vi "ShowZLUTBias.vi"(11 "Bias planes":i32) -> ()   [LabVIEW 2011]
uses:
  Main/GlobalVariables.vi
panel:
  in  "Bead index":i32
  out "Bias":sgl[](graph)
  out "All beads bias":sgl[][](graph)
  in  "Close dialog":bool
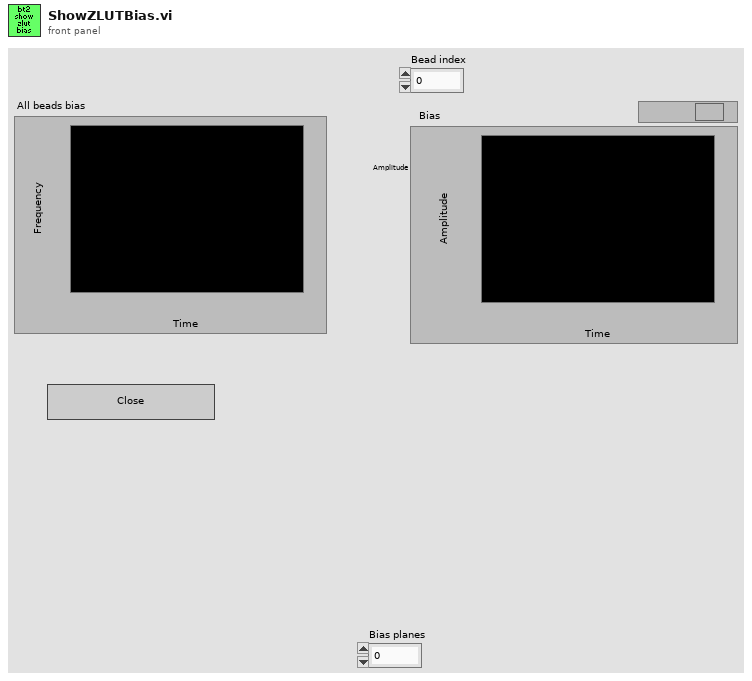
[diagram p1: front panel]
types:
  T1 = typedef "MeasureConfigType.ctl" = cluster{"Bead locations":cluster{"X":i32, "Y":i32}[], "ROI":i32, "Experiment base path":path, "Image output subdir":string, "Output mode":T2, "Traces output subdir":string, "QTrk Settings":T3, "Tracking Config":T4, "Experiment Name":string, "Program":T7, "ZLUT":sgl[][][], "Camera settings":T14, "Experiment Script":string, "Max frames in memory":i32, "Save traces as binary":bool, "Pixel Calibration Gain Image":string, "Pixel Calibration Offset Image":string, "Use pixel calibration images":bool, "Internal camera settings":string, "Trace write interval":i32}
  T2 = typedef "MeasureConfigOutputMode.ctl" = enum16{"None", "Track", "SaveImages"}
  T3 = typedef "QTrkSettings.ctl" = cluster{"Image width":i32, "Image height":i32, "Number of threads (CPU based)":i32, "CUDA Device":i32, "COM Background correction factor":sgl, "ZLUT MinRadius":sgl, "ZLUT Radial sample density":sgl, "ZLUT Angular sample density":sgl, "ZLUT ROI Coverage":sgl, "QI Iterations":i32, "QI MinRadius":sgl, "QI Radial sample density":sgl, "QI Angular sample density":sgl, "QI ROI Coverage":sgl, "QI Angular Step \nIteration Factor":sgl, "XCOR Profile Length":i32, "XCOR Profile Width":i32, "XCOR Iterations":i32, "Gaussian 2D Fit Iterations":i32, "Gaussian 2D Sigma (pixels)":sgl, "Downsample":i32}
  T4 = typedef "TrackingConfigType.ctl" = cluster{"Number of steps":i32, "ZLUT stepsize (um)":sgl, "Z correction factor":sgl, "Start piezo Z (um)":sgl, "Pixel size (nm)":sgl, "2D Localization Type":T5, "Z Command (None)":T6, "Z Piezo scale":bool, "ZLUT Building\nimages per frame":i32, "ZLUT Bias correction planes":i32}
  T5 = typedef "QTrkLocalizationType.ctl" = enum16{"Center-of-Mass", "1D Cross-Correlation", "Quadrant Interpolation", "Gaussian 2D MLE", "QI + ZLUTAlign", "ZLUTAlign", "QI + FourierLUT"}
  T6 = typedef "QTrkZCommandType.ctl" = enum16{"Nothing", "ComputeZ", "BuildRadialZLUT", "BuildImageZLUT", "RadialZLUT+ImageZLUT"}
  T7 = typedef "ExperimentProgramType.ctl" = cluster{"Commands":T8[], "Motor Axis accuracy conditions":T11, "Axis flags":T13}
  T8 = typedef "ExProgCommandType.ctl" = cluster{"cmd":T9, "axis":T10, "value/pos":dbl, "speed":dbl, "name":string}
  T9 = typedef "ExProgCommandEnumType.ctl" = enum16{"wait", "move", "event", "idle", "when", "section", "stop"}
  T10 = typedef "MotorAxisEnum.ctl" = enum16{"no axis", "magrot", "magpos", "px", "py", "pz", "camx", "camy"}
  T11 = typedef "MotorPosType.ctl" = cluster{"Magnet Z":dbl, "Magnet rotation":dbl, "Camera":T12, "Piezo XY":T12, "Piezo Z":dbl}
  T12 = typedef "XYf.ctl" = cluster{"X":sgl, "Y":sgl}
  T13 = typedef "MotorPosFlagsType.ctl" = cluster{"Magnet Z":bool, "Magnet rotation":bool, "Camera":cluster{"X":bool, "Y":bool}, "Piezo XY":cluster{"X":bool, "Y":bool}, "Piezo Z":bool}
  T14 = typedef "GenericCameraConfigType.ctl" = cluster{"Framerate (Hz)":i32, "Exposure time (us)":i32, "Image size":cluster{"Width":i32, "Height":i32}, "Number of buffers":i32}
  T15 = typedef "QTrkInstance.ctl" = cluster{"QTrk Pointer":u64}
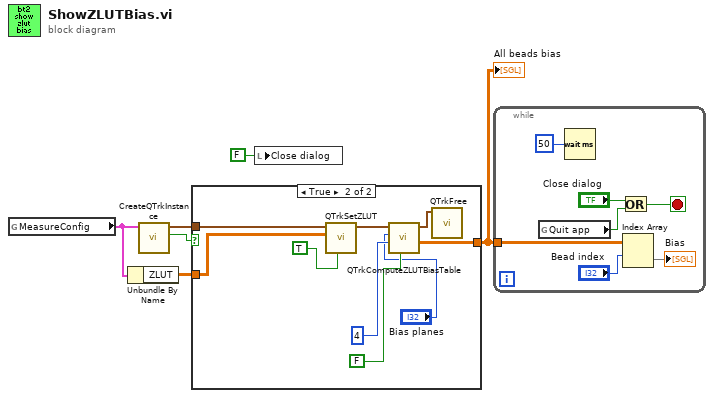
[diagram p0: block diagram]
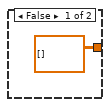
[diagram p2: hidden frame]
diagram:
  n1 = global read "GlobalVariables.vi" "MeasureConfig"() -> (w3:T1)
  n2 = Unbundle By Name(w3) -> ("ZLUT"=w4:sgl[][][])
  n3 = call "CreateQTrkInstance.vi"("MeasureConfig"=w3) -> ("Go-ahead?"=w6:bool, "QTrk Instance"=w5:T15)  [unwired: 9 in]
  n4 = case shown="True" w6 {
    tunnel: w5 -> [_ w16]
    tunnel: w4 -> [_ w13]
    tunnel: [sgl[][] [] ("Bias correction table") w9] -> w2
    frame False {
    }
    frame True {
      n5 = call "QTrkSetZLUT.vi"("Normalize LUT"=TRUE, "ZLUT"=w13, "QTrk Instance"=w16) -> ("QTrk Instance"=w14:T15)  [unwired: 7 in, 1 out]
      n6 = call "QTrkComputeZLUTBiasTable.vi"("Use spline interpolation?"=FALSE, "smpPerPixel"=4, "bias planes"="Bias planes", "QTrk Instance"=w14) -> ("Bias correction table"=w9:sgl[][], "QTrk Instance"=w10:T15)  [unwired: 5 in, 1 out]
      n7 = call "QTrkFree.vi"("QTrk Instance"=w10) -> ()  [unwired: 6 in, 1 out]
    }
  }
  "All beads bias" <- w2
  n8 = local write "Close dialog"(FALSE ("Close dialog")) -> ()
  n9 = while {
    tunnel: w2 -> [w19]
    stop <- w21 stop-if-true
    n10 = global read "GlobalVariables.vi" "Quit app"() -> (w22:bool)
    n11 = Wait (ms)(milliseconds to wait=u32 50) -> ()  [unwired: 1 out]
    n12 = Or(x="Close dialog", y=w22) -> (x .or. y?=w21:bool)
    n13 = Index Array(array=w19, index (row)="Bead index") -> (element=→"Bias":sgl[])  [unwired: 1 in]
  }
